vi "Archiver.vi"() -> ()   [LabVIEW 2009]
uses:
  HDF5/Clients/H5F-File/H5F_ACC.ctl
panel:
  in  "Ratio Count":i32=20
  in  "Fringes Count":i32=200
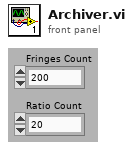
[diagram p1: front panel]
types:
  T1 = typedef "H5F_ACC.ctl" = enum16{"RDONLY", "RDWR", "TRUNC", "EXCL", "DEBUG", "CREAT"}
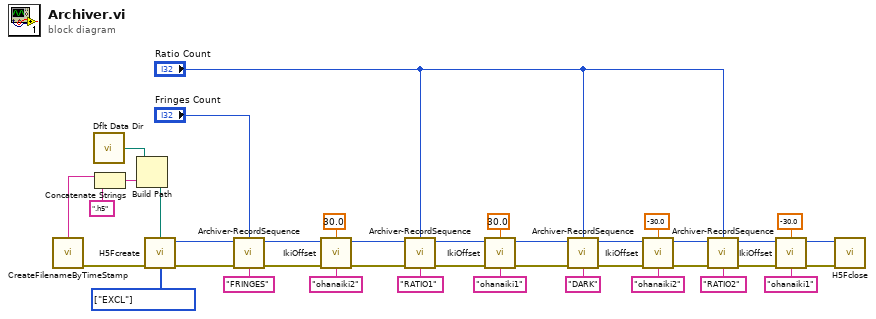
[diagram p0: block diagram]
diagram:
  w31 = T1[] [enum."EXCL"] items=["RDONLY", "RDWR", "TRUNC", "EXCL", "DEBUG", "CREAT"] ("flags")
  n1 = call "CreateFilenameByTimeStamp.vi"() -> ("Filename"=w3:string, "error out"=w27:errorcluster)  [unwired: 8 in]
  n2 = call <vilib>:"Dflt Data Dir.vi"() -> ("App:Default Data Directory"=w26:path)
  n3 = Concatenate Strings(w3, ".h5" ("string")) -> (w2:string)
  n4 = Build Path(base path=w26, name or relative path=w2) -> (appended path=w25:path)
  n5 = call "H5Fcreate.vi"("filename"=w25, "flags"=w31, "error in (no error)"=w27) -> ("file_id"=w9:i32, "error out"=w30:errorcluster)  [unwired: 5 in]
  n6 = call "Archiver-RecordSequence.vi"("Count"="Fringes Count", "file_id"=w9, "name"="FRINGES", "error in (no error)"=w30) -> ("error out"=w23:errorcluster)  [unwired: 5 in]
  n7 = call "IkiOffset.vi"("Y offset"=30.0, "Iki Name"="ohanaiki2", "error in (no error)"=w23) -> ("error out"=w20:errorcluster)  [unwired: 6 in]
  n8 = call "Archiver-RecordSequence.vi"("Count"="Ratio Count", "file_id"=w9, "name"="RATIO1", "error in (no error)"=w20) -> ("error out"=w17:errorcluster)  [unwired: 5 in]
  n9 = call "IkiOffset.vi"("Y offset"=30.0, "Iki Name"="ohanaiki1", "error in (no error)"=w17) -> ("error out"=w15:errorcluster)  [unwired: 6 in]
  n10 = call "Archiver-RecordSequence.vi"("Count"="Ratio Count", "file_id"=w9, "name"="DARK", "error in (no error)"=w15) -> ("error out"=w12:errorcluster)  [unwired: 5 in]
  n11 = call "IkiOffset.vi"("Y offset"=-30.0, "Iki Name"="ohanaiki2", "error in (no error)"=w12) -> ("error out"=w10:errorcluster)  [unwired: 6 in]
  n12 = call "Archiver-RecordSequence.vi"("Count"="Ratio Count", "file_id"=w9, "name"="RATIO2", "error in (no error)"=w10) -> ("error out"=w4:errorcluster)  [unwired: 5 in]
  n13 = call "IkiOffset.vi"("Y offset"=-30.0, "Iki Name"="ohanaiki1", "error in (no error)"=w4) -> ("error out"=w5:errorcluster)  [unwired: 6 in]
  n14 = call "H5Fclose.vi"("error in (no error)"=w5, "file_id"=w9) -> ()  [unwired: 8 in, 2 out]
